vi "Get Size.vi"(3 "WavBuf":refnum<class "WavBuf.lvclass">) -> (1 "Buffer Size Out":i32)   [LabVIEW 2025, in "WavBuf.lvclass"]
uses:
  WavBuf.lvclass
  WavBuf.lvclass/WavBuf.ctl
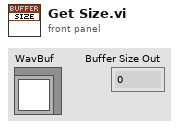
[diagram p1: front panel]
types:
  T1 = typedef "Ref_DVR_Buffer.ctl" = refnum<data-value>
  T2 = typedef "Waveform_Data.ctl" = waveform(dbl)
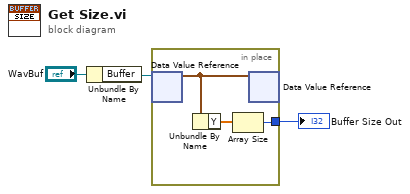
[diagram p0: block diagram]
diagram:
  n1 = Unbundle By Name("WavBuf") -> ("Buffer"=w1:T1)
  n2 = in-place {
    in-place-border: [w4] -> w2
    n3 = in-place-dvr #1(w1) -> (w5:T2)  [unwired: 1 out]
    n4 = Unbundle By Name(w5) -> ("Y"=w6:dbl[])
    n5 = Array Size(array=w6) -> (size(s)=w4:i32)
    n6 = in-place-dvr #1(w5) -> ()  [unwired: 2 out]
  }
  "Buffer Size Out" <- w2
